vi "RSZVB Error Query.vi"(8 "error in (no error)":errorcluster {"code" format="%.0x"}, 11 "VISA session":refnum<visa-resource-name>) -> (0 "error out":errorcluster {"code" format="%.0x"}, 1 "Error Message":string, 2 "Error":i32, 3 "dup VISA session":refnum<visa-resource-name>)   [LabVIEW 2015]
doc: "This VI reads an error code and a message from the instrument's error queue.\n\nNote:\nThis VI is called automatically by most driver VIs so it is not usually necessary to call this in an application."
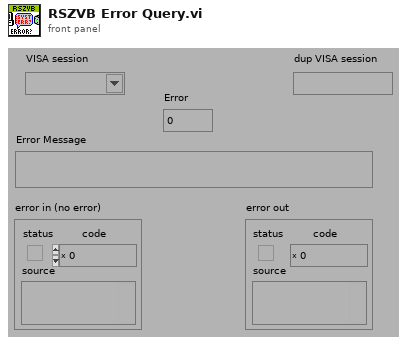
[diagram p1: front panel]
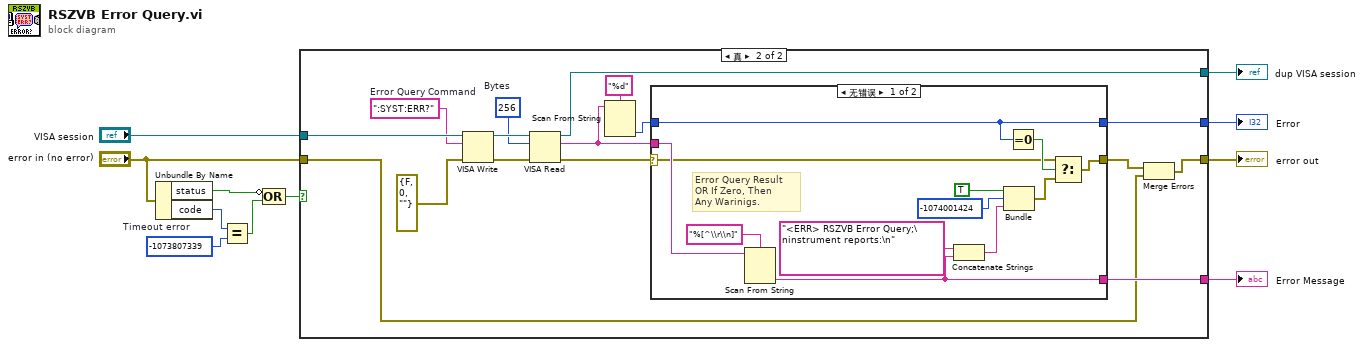
[diagram p0: block diagram]
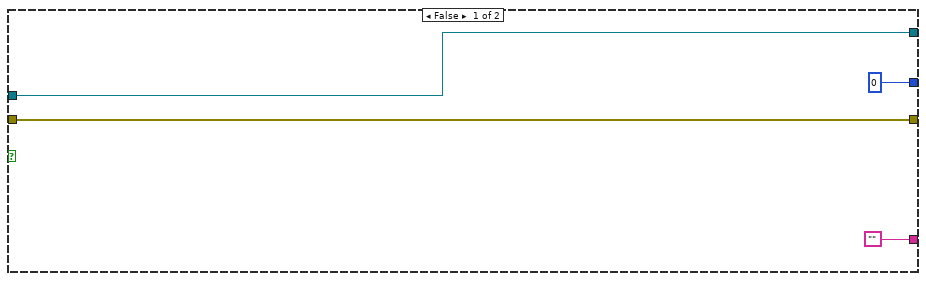
[diagram p2: hidden frame]
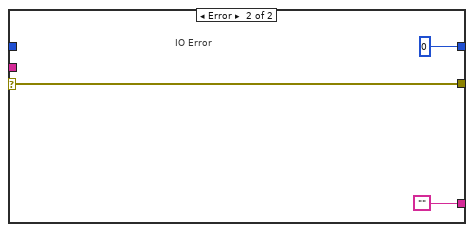
[diagram p3: hidden frame]
diagram:
  w4 = -1073807339  # Timeout error
  n1 = Unbundle By Name("error in (no error)") -> ("status"=w5:bool, "code"=w3:i32)
  n2 = Equal?(x=w3, y=w4) -> (x = y?=w2:bool)
  n3 = Compound Arithmetic op=OR(invert w5, w2) -> (w1:bool)
  n4 = case shown="真" w1 {
    tunnel: ["" w31] -> w11
    tunnel: [0 w30] -> w10
    tunnel: [w15 w29] -> w9
    tunnel: "VISA session" -> [w15 w28]
    tunnel: "error in (no error)" -> [w12 w21]
    tunnel: [w12 w20] -> w7
    frame False {
    }
    frame True {
      w26 = u32 256  # Bytes
      w24 = ":SYST:ERR?"  # Error Query Command
      n5 = VISA Write(VISA resource name=w28, write buffer=w24, error in (no error)=errorcluster {"status"=FALSE, "code"=0, "source"=""}) -> (VISA resource name out=w27:refnum<visa-resource-name>, error out=w25:errorcluster)  [unwired: 1 out]
      n6 = VISA Read(VISA resource name=w27, byte count=w26, error in (no error)=w25) -> (VISA resource name out=w29:refnum<visa-resource-name>, read buffer=w19:string, error out=w16:errorcluster)  [unwired: 1 out]
      n7 = Scan From String(format string="%d", input string=w19) -> (output 1=w17:i32)  [unwired: 3 in, 3 out]
      n8 = case shown="无错误" w16 {
        selector: w16 -> [w32 w44]
        tunnel: w19 -> [w34 _]
        tunnel: [w39 w44] -> w22
        tunnel: [w35 ""] -> w31
        tunnel: [w33 0] -> w30
        tunnel: w17 -> [w33 _]
        frame No Error {
          # "Error Query Result\nOR If Zero, Then\nAny Warinigs."
          n9 = Scan From String(format string="%[^\\r\\n]", input string=w34) -> (output 1=w35:string)  [unwired: 3 in, 3 out]
          n10 = Concatenate Strings("<ERR> RSZVB Error Query;\ninstrument reports:\n" ("Source"), w35) -> (w41:string)
          n11 = Bundle("Status"=TRUE, "Code"=-1074001424, w41) -> (w40:cluster{"Status":bool, "Code":i32, string})  [unwired: 1 in]
          n12 = Equal To 0?(x=w33) -> (x = 0?=w37:bool)
          n13 = Select(t=w32, s=w37, f=w40) -> (s? t:f=w39:errorcluster)
        }
        frame Error {
          # "IO Error"
        }
      }
      n14 = Merge Errors(w22, w21) -> (w20:errorcluster)
    }
  }
  "Error Message" <- w11
  "Error" <- w10
  "dup VISA session" <- w9
  "error out" <- w7
